vi "Query.vi"(8 "error in (no error)":errorcluster, 10 "Service":T1, 11 "MicronCLI in":refnum<class "MicronCLI.lvclass">) -> (0 "error out":errorcluster, 2 "ConnectionString":string, 3 "MicronCLI out":refnum<class "MicronCLI.lvclass">)   [LabVIEW 2019, in "MicronCLI.lvclass"]
uses:
  MicronCLI.lvclass
  Typedefs/ServiceDetails.ctl
  MicronCLI.lvclass/MicronCLI.ctl
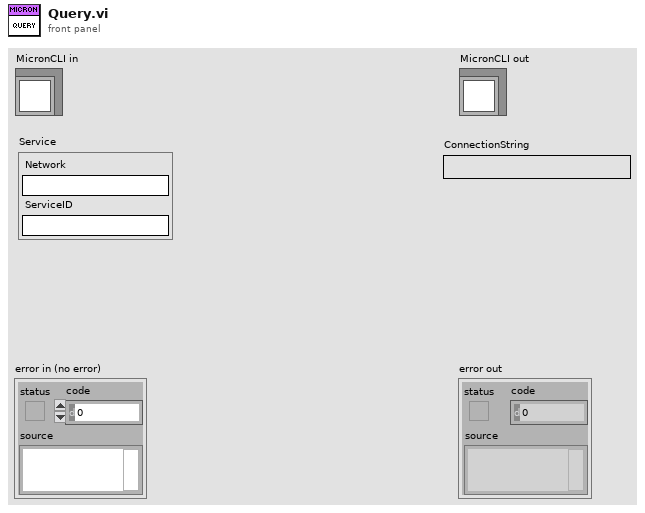
[diagram p1: front panel]
types:
  T1 = typedef "MicronCLI.lvclass/ServiceDetails.ctl" = cluster{"Network":string, "ServiceID":string}
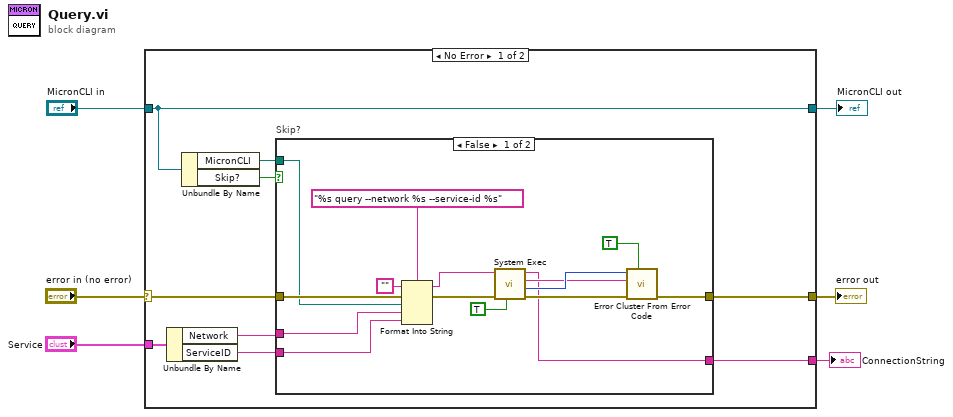
[diagram p0: block diagram]
diagram:
  n1 = case shown="No Error" "error in (no error)" {
    selector: "error in (no error)" -> [w15 w33]
    tunnel: [w12 w33] -> w5
    tunnel: [w14 w32] -> w3
    tunnel: "MicronCLI in" -> [w14 w32]
    tunnel: [w11 _] -> w2
    tunnel: "Service" -> [w9 _]
    frame No Error {
      n2 = Unbundle By Name(w9) -> ("Network"=w8:string, "ServiceID"=w7:string)
      n3 = Unbundle By Name(w14) -> ("MicronCLI"=w13:path, "Skip?"=w10:bool)
      n4 = case "Skip?" shown="False" w10 {
        tunnel: w15 -> [w30 w31]
        tunnel: w13 -> [w26 _]
        tunnel: [w22 w31] -> w12
        tunnel: [w18 _] -> w11
        tunnel: w8 -> [w17 _]
        tunnel: w7 -> [w16 _]
        frame False {
          n5 = Format Into String(format string="%s query --network %s --service-id %s", initial string="", error in=w30, w26, w17, w16) -> (resulting string=w24:string, error out=w28:errorcluster)
          n6 = call <vilib>:"System Exec.vi"("run minimized? (F)"=TRUE, "error in (no error)"=w28, "command line"=w24) -> ("error out"=w29:errorcluster, "return code"=w21:i32, "standard error"=w20:string, "standard output"=w18:string)  [unwired: 5 in]
          n7 = call <vilib>:"Error Cluster From Error Code.vi"("show call chain? (False)"=TRUE, "error in (no error)"=w29, "error message (\"\")"=w20, "error code (0)"=w21) -> ("error out"=w22:errorcluster)  [unwired: 5 in]
        }
        frame True {
        }
      }
    }
    frame Error {
    }
  }
  "error out" <- w5
  "MicronCLI out" <- w3
  "ConnectionString" <- w2
